vi "update available parameters.vi"(9 "inventory":T1, 10 "Device selection":refnum<vi>, 11 "Available parameters":refnum<vi>) -> ()   [LabVIEW 2016]
uses:
  inventory type def.ctl
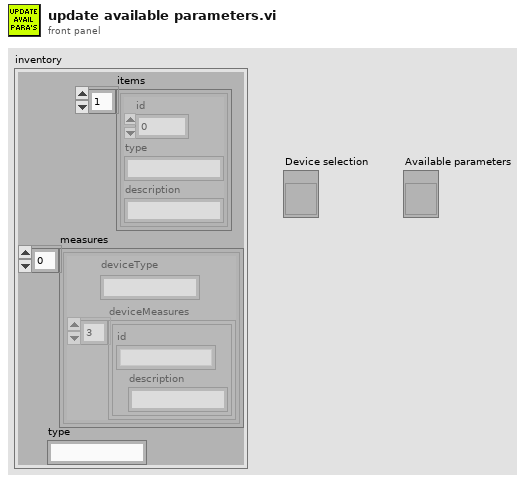
[diagram p1: front panel]
types:
  T1 = typedef "inventory type def.ctl" = cluster{"items":cluster{"id":u8, "type":string, "description":string}[], "measures":cluster{"deviceType":string, "deviceMeasures":cluster{"id":string, "description":string}[]}[], "type":string}
  T2 = cluster{"id":u8, "type":string, "description":string}[]
  T3 = cluster{"id":u8, "type":string, "description":string}
  T4 = cluster{"deviceType":string, "deviceMeasures":cluster{"id":string, "description":string}[]}[]
  T5 = cluster{"deviceType":string, "deviceMeasures":cluster{"id":string, "description":string}[]}
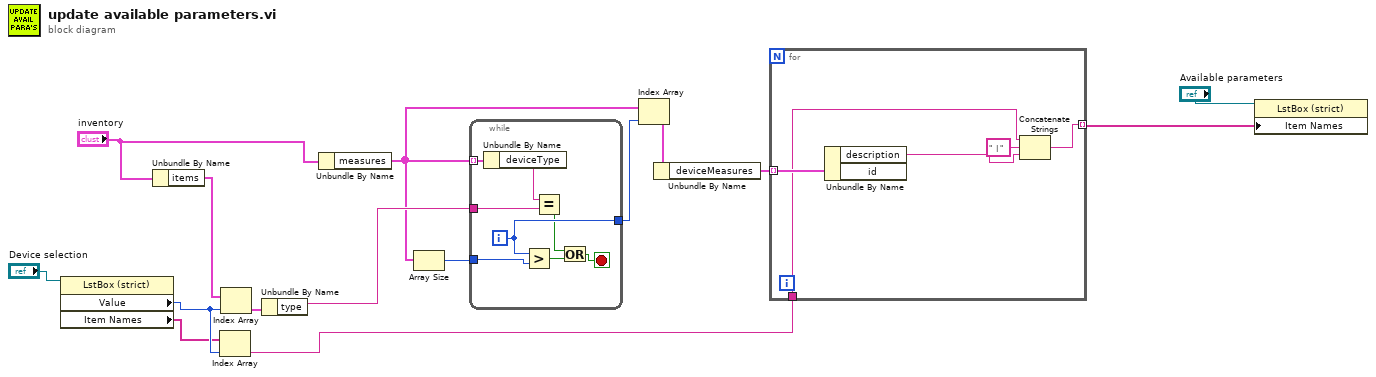
[diagram p0: block diagram]
diagram:
  n1 = property class="LstBox (strict)"(reference="Device selection") -> ("Value"=w9:i32, "Item Names"=w8:string[])  [unwired: 1 in, 2 out]
  n2 = Unbundle By Name("inventory") -> ("items"=w10:T2)
  n3 = Index Array(array=w8, index=w9) -> (element=w7:string)
  n4 = Index Array(array=w10, index=w9) -> (element=w13:T3)
  n5 = Unbundle By Name(w13) -> ("type"=w6:string)
  n6 = Unbundle By Name("inventory") -> ("measures"=w4:T4)
  n7 = Array Size(array=w4) -> (size(s)=w5:i32)
  n8 = while {
    tunnel: w4 -> [w23] mode=indexing
    tunnel: w6 -> [w21]
    tunnel: [w20] -> w3
    tunnel: w5 -> [w19]
    i -> [w20]
    stop <- w17 stop-if-true
    n9 = Unbundle By Name(w23) -> ("deviceType"=w22:string)
    n10 = Greater?(x=w20, y=w19) -> (0:w18:bool)
    n11 = Equal?(x=w22, y=w21) -> (x = y?=w16:bool)
    n12 = Or(x=w16, y=w18) -> (x .or. y?=w17:bool)
  }
  n13 = Index Array(array=w4, index=w3) -> (element=w2:T5)
  n14 = Unbundle By Name(w2) -> ("deviceMeasures"=w1:cluster{"id":string, "description":string}[])
  n15 = for {
    tunnel: [w27] -> w12 mode=indexing
    tunnel: w7 -> [w24]
    tunnel: w1 -> [w26] mode=indexing
    n16 = Unbundle By Name(w26) -> ("description"=w25:string)  [unwired: 1 out]
    n17 = Concatenate Strings(w24, "  | " ("string"), w25) -> (w27:string)
  }
  n18 = property class="LstBox (strict)"(reference="Available parameters", "Item Names"=w12) -> ()  [unwired: 1 in, 2 out]
